vi "Is stroker Moving.vi"(0 "Connected":bool, 7 "Position":dbl) -> (3 "Decrease":bool, 4 "Known":bool, 6 "Changing":bool, 8 "Increasing":bool, 10 "Increase":T1, 15 "Decrease":T1)   [LabVIEW 2011]
uses:
  Measurments Handling/Status Digitalish.ctl
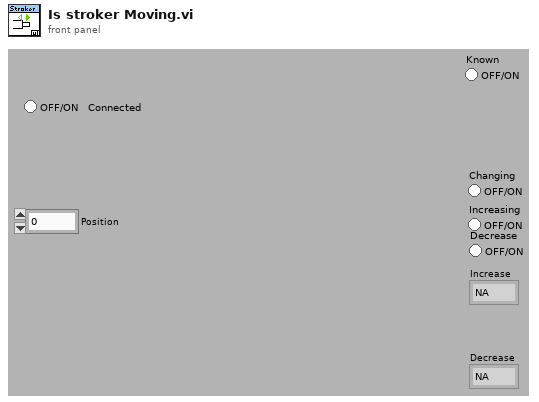
[diagram p1: front panel]
types:
  T1 = typedef "Status Digitalish.ctl" = enum16{"NA", "False", "True"}
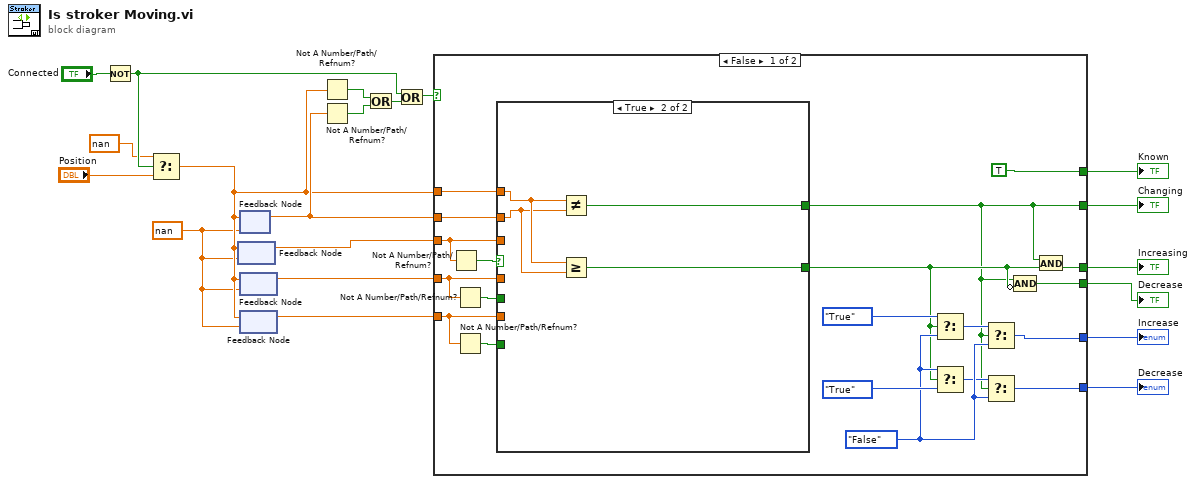
[diagram p0: block diagram]
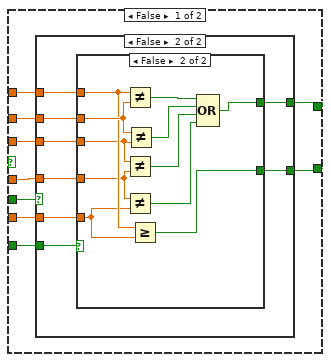
[diagram p2: hidden frame]
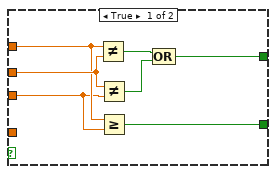
[diagram p3: hidden frame]
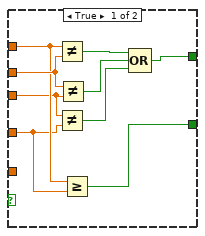
[diagram p4: hidden frame]
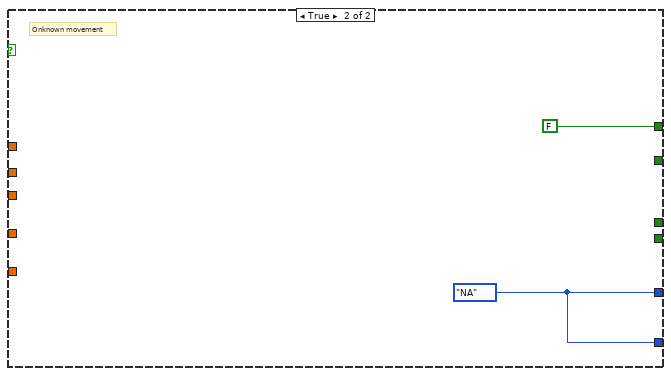
[diagram p5: hidden frame]
diagram:
  w2 = nan ("Position")
  n1 = Not(x="Connected") -> (.not. x?=w4:bool)
  n2 = Select(t=nan, s=w4, f="Position") -> (s? t:f=w5:dbl)
  n3 = feedback-in #1(w5) -> ()
  n4 = feedback #1(w2) -> (w20:dbl)
  n5 = feedback-in #2(w5) -> ()
  n6 = feedback #2(w2) -> (w19:dbl)
  n7 = feedback #3(w2) -> (w7:dbl)
  n8 = feedback-in #3(w5) -> ()
  n9 = feedback #4(w2) -> (w6:dbl)
  n10 = feedback-in #4(w5) -> ()
  n11 = Not A Number/Path/Refnum?(number/path/refnum=w5) -> (NaN/Path/Refnum?=w18:bool)
  n12 = Not A Number/Path/Refnum?(number/path/refnum=w19) -> (NaN/Path/Refnum?=w17:bool)
  n13 = Or(x=w18, y=w17) -> (x .or. y?=w16:bool)
  n14 = Or(x=w4, y=w16) -> (x .or. y?=w12:bool)
  n15 = case shown="False" w12 {
    tunnel: w20 -> [w38 _]
    tunnel: w19 -> [w40 _]
    tunnel: w5 -> [w39 _]
    tunnel: [w21 _] -> w15
    tunnel: [w22 _] -> w14
    tunnel: [TRUE FALSE] -> w13
    tunnel: [w30 w89] -> w10
    tunnel: [w29 w89] -> w9
    tunnel: w7 -> [w27 _]
    tunnel: w6 -> [w25 _]
    tunnel: [w23 _] -> w1
    frame False {
      w33 = Status_Digitalish."False" ("Status")
      n16 = Not A Number/Path/Refnum?(number/path/refnum=w38) -> (NaN/Path/Refnum?=w37:bool)
      n17 = Not A Number/Path/Refnum?(number/path/refnum=w27) -> (NaN/Path/Refnum?=w28:bool)
      n18 = Not A Number/Path/Refnum?(number/path/refnum=w25) -> (NaN/Path/Refnum?=w26:bool)
      n19 = case shown="True" w37 {
        tunnel: w40 -> [w49 w87]
        tunnel: w39 -> [w48 w88]
        tunnel: w38 -> [w47 _]
        tunnel: [w46 w86] -> w21
        tunnel: [w45 w85] -> w24
        tunnel: w28 -> [w44 _]
        tunnel: w27 -> [w43 _]
        tunnel: w25 -> [w42 _]
        tunnel: w26 -> [w41 _]
        frame False {
          n20 = case shown="False" w44 {
            tunnel: w49 -> [w54 w64]
            tunnel: w48 -> [w53 w63]
            tunnel: w47 -> [w52 w59]
            tunnel: [w51 w62] -> w46
            tunnel: [w50 w61] -> w45
            tunnel: w43 -> [_ w60]
            tunnel: w42 -> [_ w57]
            tunnel: w41 -> [_ w58]
            frame True {
              n21 = Not Equal?(x=w53, y=w54) -> (x != y?=w56:bool)
              n22 = Not Equal?(x=w54, y=w52) -> (x != y?=w55:bool)
              n23 = Greater Or Equal?(x=w53, y=w52) -> (x >= y?=w50:bool)
              n24 = Compound Arithmetic op=OR(w56, w55) -> (w51:bool)
            }
            frame False {
              n25 = case shown="False" w58 {
                tunnel: w64 -> [w71 w82]
                tunnel: w63 -> [w70 w81]
                tunnel: [w69 w80] -> w62
                tunnel: [w68 w79] -> w61
                tunnel: w60 -> [w67 w76]
                tunnel: w59 -> [w66 w78]
                tunnel: w57 -> [_ w75]
                frame True {
                  n26 = Not Equal?(x=w70, y=w71) -> (x != y?=w73:bool)
                  n27 = Not Equal?(x=w66, y=w67) -> (x != y?=w65:bool)
                  n28 = Not Equal?(x=w71, y=w66) -> (x != y?=w72:bool)
                  n29 = Greater Or Equal?(x=w70, y=w67) -> (x >= y?=w68:bool)
                  n30 = Compound Arithmetic op=OR(w73, w72, w65) -> (w69:bool)
                }
                frame False {
                  n31 = Not Equal?(x=w81, y=w82) -> (x != y?=w84:bool)
                  n32 = Not Equal?(x=w78, y=w76) -> (x != y?=w77:bool)
                  n33 = Not Equal?(x=w76, y=w75) -> (x != y?=w74:bool)
                  n34 = Not Equal?(x=w82, y=w78) -> (x != y?=w83:bool)
                  n35 = Greater Or Equal?(x=w81, y=w75) -> (x >= y?=w79:bool)
                  n36 = Compound Arithmetic op=OR(w84, w83, w77, w74) -> (w80:bool)
                }
              }
            }
          }
        }
        frame True {
          n37 = Not Equal?(x=w88, y=w87) -> (x != y?=w86:bool)
          n38 = Greater Or Equal?(x=w88, y=w87) -> (x >= y?=w85:bool)
        }
      }
      n39 = Select(t=Status_Digitalish."True" ("Status"), s=w24, f=w33) -> (s? t:f=w32:T1)
      n40 = Select(t=w33, s=w24, f=Status_Digitalish."True" ("Status")) -> (s? t:f=w31:T1)
      n41 = Select(t=w32, s=w21, f=w33) -> (s? t:f=w30:T1)
      n42 = Select(t=w31, s=w21, f=w33) -> (s? t:f=w29:T1)
      n43 = Compound Arithmetic op=AND(w21, invert w24) -> (w23:bool)
      n44 = And(x=w21, y=w24) -> (x .and. y?=w22:bool)
    }
    frame True {
      w89 = Status_Digitalish."NA" ("Status")
      # "Onknown movement"
    }
  }
  "Decrease" <- w9
  "Changing" <- w15
  "Increasing" <- w14
  "Known" <- w13
  "Increase" <- w10
  "Decrease" <- w1
